vi "Rx Read Single Point.vi"(8 "error in (no error)":errorcluster, 9 "timeout [ms]":u32=100, 11 "Rx Session In":T1) -> (0 "error out":errorcluster, 2 "Data":dbl[](array[numeric]), 3 "Rx Session Out":T1)   [LabVIEW 2020, in "985x Support Addon Engine.lvlib"]
uses:
  985x Support Addon Engine.lvlib
  Types/Rx Session.ctl
  Types/FPGA Refnum.ctl
  <vilib>/xnet/xnet.llb/XNET Convert (Frame CAN to Signal).vi
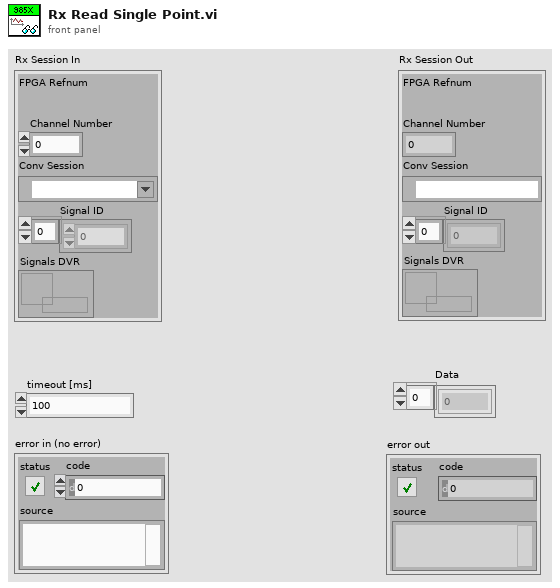
[diagram p1: front panel]
types:
  T1 = typedef "985x Support Addon Engine.lvlib/Rx Session.ctl" = cluster{"FPGA Refnum":T2, "Channel Number":u32, "Conv Session":refnum<k21>, "Signal ID":u32[], "Signals DVR":refnum<data-value>}
  T2 = typedef "985x Support Addon Engine.lvlib/FPGA Refnum.ctl" = refnum<k20>
  T3 = typedef "XNET Frame CAN.ctl" = cluster{"timestamp":timestamp, "payload":u8[], "identifier":u32, "type":T4, "extended?":bool, "echo?":bool}
  T4 = typedef "XNET Frame Type CAN.ctl" = u8
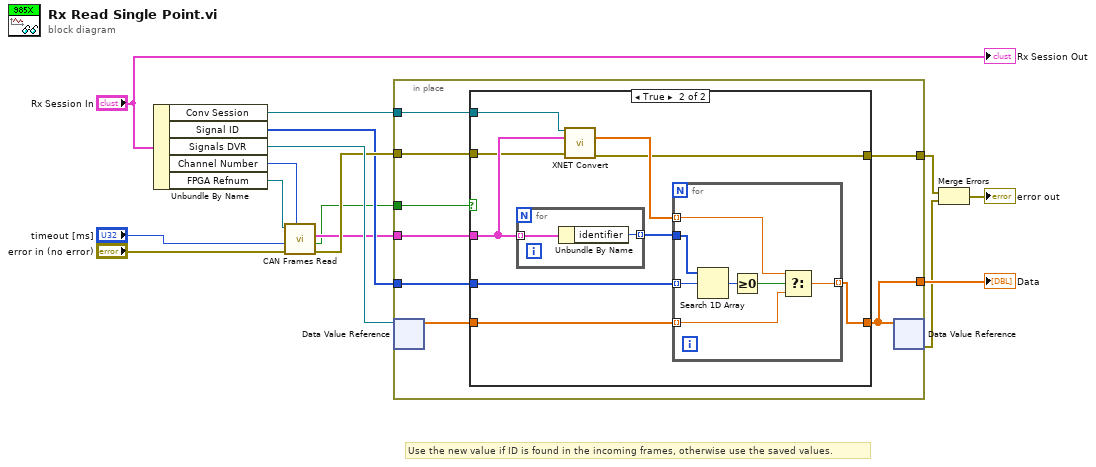
[diagram p0: block diagram]
diagram:
  # "Use the new value if ID is found in the incoming frames, otherwise use the saved values."
  n1 = Unbundle By Name("Rx Session In") -> ("Conv Session"=w12:refnum<k21>, "Signal ID"=w10:u32[], "Signals DVR"=w13:refnum<data-value>, "Channel Number"=w2:u32, "FPGA Refnum"=w1:T2)
  n2 = call "CAN Frames Read.vi"("Channel Number"=w2, "error in (no error)"="error in (no error)", "timeout [ms]"="timeout [ms]", "FPGA Refnum"=w1) -> ("error out"=w11:errorcluster, "Valid"=w4:bool, "Frames"=w5:T3[])  [unwired: 5 in]
  n3 = in-place {
    in-place-border: w10 -> [w22]
    in-place-border: [w21] -> w14
    in-place-border: w5 -> [w18]
    in-place-border: w12 -> [w20]
    in-place-border: w11 -> [w19]
    in-place-border: [w17] -> w9
    in-place-border: w4 -> [w16]
    n4 = in-place-dvr #1(w13) -> (w23:dbl[])  [unwired: 1 out]
    n5 = case shown="True" w16 {
      tunnel: w23 -> [w25 w34]
      tunnel: w22 -> [_ w33]
      tunnel: [w25 w32] -> w21
      tunnel: w20 -> [_ w31]
      tunnel: w18 -> [_ w30]
      tunnel: w19 -> [w24 w29]
      tunnel: [w24 w26] -> w17
      frame False {
      }
      frame True {
        n6 = for {
          tunnel: w30 -> [w36] mode=indexing
          tunnel: [w35] -> w28 mode=indexing
          n7 = Unbundle By Name(w36) -> ("identifier"=w35:u32)
        }
        n8 = call-poly <vilib>:"XNET Convert.vi"("session in"=w31, "frame data"=w30, "error in (no error)"=w29) -> ("signal data"=w27:dbl[], "error out"=w26:errorcluster)  [unwired: 11 out]
        n9 = for {
          tunnel: w34 -> [w38] mode=indexing
          tunnel: w33 -> [w42] mode=indexing
          tunnel: w28 -> [w43]
          tunnel: w27 -> [w39] mode=indexing
          tunnel: [w37] -> w32 mode=indexing
          n10 = Search 1D Array(1D array=w43, element=w42) -> (index of element=w41:i32)  [unwired: 1 in]
          n11 = Greater Or Equal To 0?(x=w41) -> (x >= 0?=w40:bool)
          n12 = Select(t=w39, s=w40, f=w38) -> (s? t:f=w37:dbl)
        }
      }
    }
    n13 = in-place-dvr #1(w21) -> (w8:errorcluster)  [unwired: 1 out]
  }
  "Data" <- w14
  n14 = Merge Errors(w9, w8) -> (→"error out":errorcluster)
  "Rx Session Out" <- "Rx Session In"
